vi "set step.vi"(8 "error in (no error)":errorcluster, 10 "step":T1, 11 "Autofocus in":refnum<class "Autofocus.lvclass">) -> (0 "error out":errorcluster, 3 "Autofocus out":refnum<class "Autofocus.lvclass">)   [LabVIEW 2012, in "Autofocus.lvclass"]
uses:
  Autofocus.lvclass
  step.ctl
  Autofocus.lvclass/Autofocus.ctl
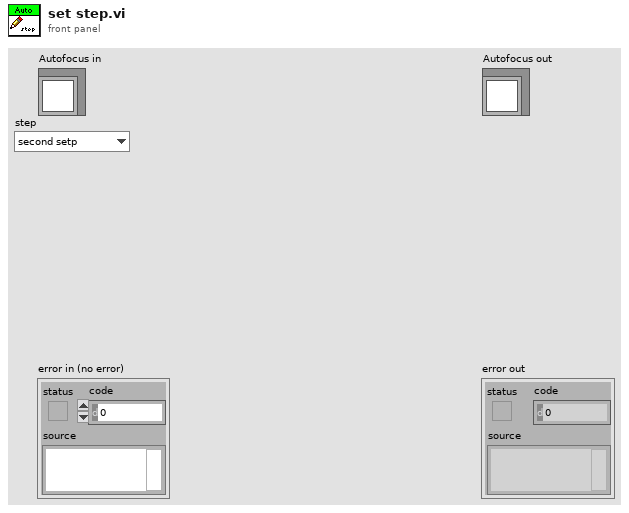
[diagram p1: front panel]
types:
  T1 = typedef "Autofocus.lvclass/step.ctl" = enum16{"second setp", "first step", "idle"}
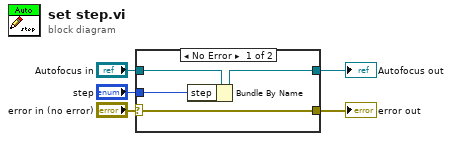
[diagram p0: block diagram]
diagram:
  n1 = case shown="No Error" "error in (no error)" {
    selector: "error in (no error)" -> [w9 w11]
    tunnel: [w9 w11] -> w4
    tunnel: [w7 w10] -> w2
    tunnel: "Autofocus in" -> [w8 w10]
    tunnel: "step" -> [w6 _]
    frame No Error {
      n2 = Bundle By Name(cluster=w8, "step"=w6) -> (w7:refnum<class "Autofocus.lvclass">)
    }
    frame Error {
    }
  }
  "error out" <- w4
  "Autofocus out" <- w2
